vi "GetLocalizedPhraseLowLevel.vi"(7 "Dictionary":T1, 8 "error in (no error)":errorcluster, 10 "Target Language":string, 11 "Key":string) -> (0 "error out":errorcluster, 2 "Key Present?":bool, 3 "Localized Phrase":string)   [LabVIEW 2020]
uses:
  Dictionary--Cluster.ctl
  Font -- Cluster.ctl
  Phrase Dictionary Entry -- Cluster.ctl
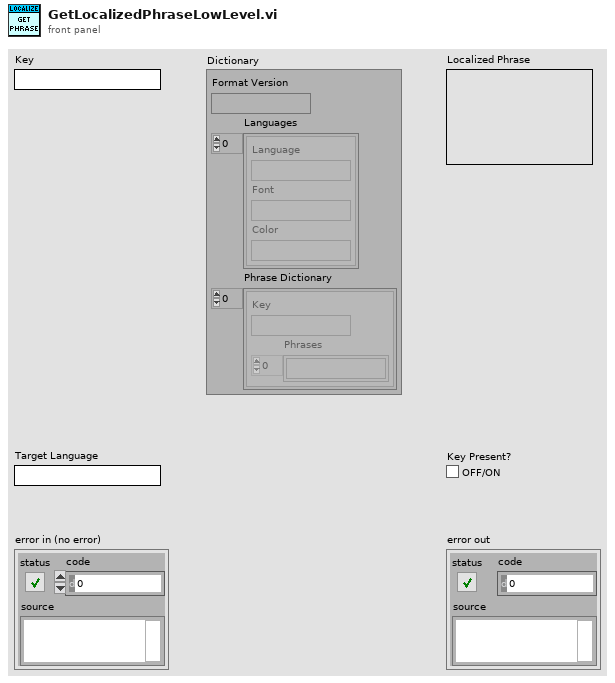
[diagram p1: front panel]
types:
  T1 = typedef "Dictionary--Cluster.ctl" = cluster{"Format Version":string, "Languages":T2[], "Phrase Dictionary":T3[]}
  T2 = typedef "Font -- Cluster.ctl" = cluster{"Language":string, "Font":string, "Color":string}
  T3 = typedef "Phrase Dictionary Entry -- Cluster.ctl" = cluster{"Key":string, "Phrases":string[]}
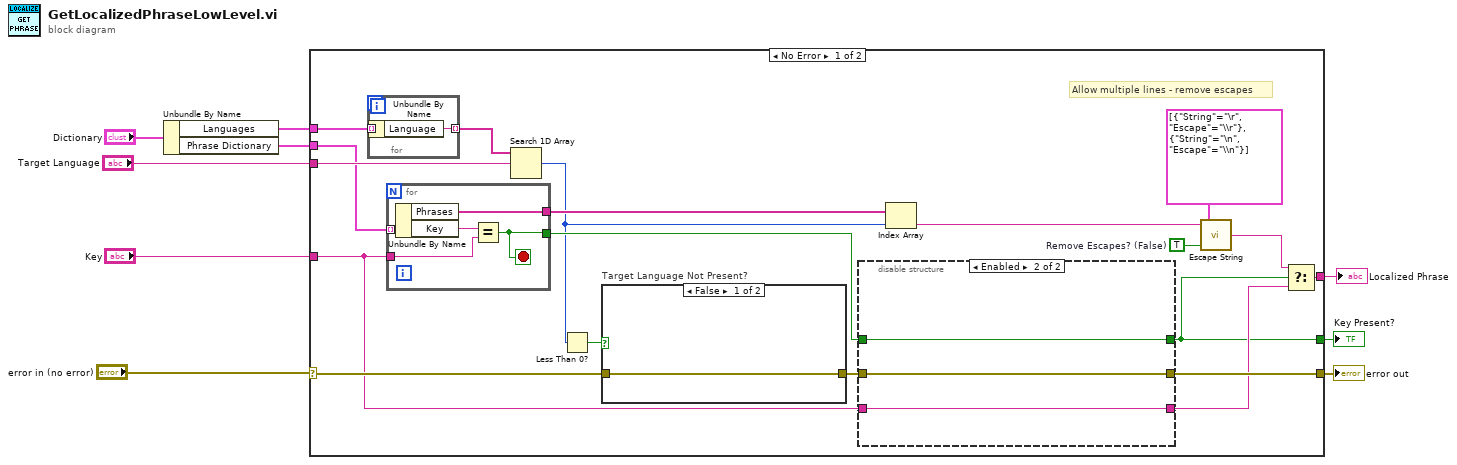
[diagram p0: block diagram]
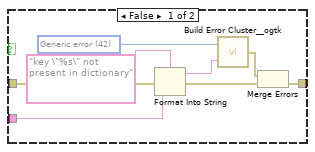
[diagram p3: hidden frame]
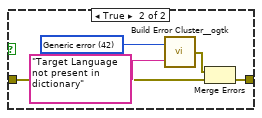
[diagram p4: hidden frame]
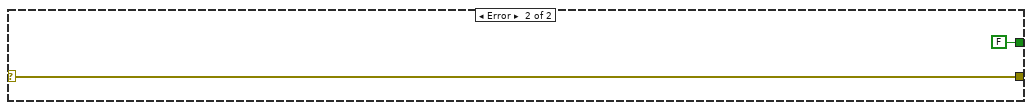
[diagram p5: hidden frame]
diagram:
  n1 = Unbundle By Name("Dictionary") -> ("Languages"=w4:T2[], "Phrase Dictionary"=w2:T3[])
  n2 = case shown="No Error" "error in (no error)" {
    selector: "error in (no error)" -> [w24 w59]
    tunnel: w4 -> [w14 _]
    tunnel: [w16 _] -> w9
    tunnel: [w17 w59] -> w8
    tunnel: "Target Language" -> [w23 _]
    tunnel: "Key" -> [w15 _]
    tunnel: w2 -> [w18 _]
    tunnel: [w10 FALSE] -> w1
    frame No Error {
      w26 = TRUE  # Remove Escapes? (False)
      # "Allow multiple lines - remove escapes"
      n3 = for {
        tunnel: w14 -> [w46] mode=indexing
        tunnel: [w45] -> w13 mode=indexing
        n4 = Unbundle By Name(w46) -> ("Language"=w45:string)
      }
      n5 = for {
        tunnel: w18 -> [w51] mode=indexing
        tunnel: w15 -> [w49]
        tunnel: [w48] -> w21
        tunnel: [w47] -> w22
        stop <- w48 stop-if-true
        n6 = Unbundle By Name(w51) -> ("Phrases"=w47:string[], "Key"=w50:string)
        n7 = Equal?(x=w50, y=w49) -> (x = y?=w48:bool)
      }
      n8 = Search 1D Array(1D array=w13, element=w23) -> (index of element=w20:i32)  [unwired: 1 in]
      n9 = Less Than 0?(x=w20) -> (x < 0?=w28:bool)
      n10 = case "Target Language Not Present?" shown="False" w28 {
        tunnel: w24 -> [w52 w54]
        tunnel: [w52 w53] -> w27
        frame False {
        }
        frame True {
          w57 = 42 items=["No error", "Argument error", "Memory is full", "Out of zone", "End of file", "File already open", "Generic file I/O error", "File not found", "File permission error", "Disk is full", "Duplicate path", "Too many files open", "System feature not enabled", "Resource file not found", "Cannot add resource", "Resource not found", "Image not found", "Image memory error", "Pen does not exist", "Config type invalid", "Config token not found", "Config parse error", "Config memory error", "Bad external code format", "Bad external code offset", "External code not present", "Null window", "Destroy window error", "Null menu", "Print aborted", "Bad print record", "Print driver error", "Windows error during printing", "Memory error during printing", "Print dialog error", "Generic print error", "Invalid device refnum", "Device not found", "Device parameter error", "Device unit error", "Cannot open device", "Device call aborted", "Generic error", "Cancelled by user", "Object ID too low", "Object ID too high", "Object not in heap", "Unknown heap", "Unknown object (invalid DefProc)", "Unknown object (DefProc not in table)", "Message out of range", "Invalid (null) method", "Unknown message", "Manager call not supported", "Bad address", "Network operation in progress", "Network operation timed out", "Connection is busy", "Network attribute not supported", "Network error", "Address in use", "System out of memory", "Connection aborted", "Connection refused", "Not connected", "Already connected", "Connection closed", "Initialization error (interapplication manager)", "Bad occurrence", "Wait on unbound occurrence handler", "Occurrence queue overflow", "Datalog type conflict", "Unused", "Unrecognized type (interapplication manager)", "Memory corrupt", "Failed to make temporary DLL", "Old CIN version", "Drag socket not found", "Failed to load drop-object", "Failed to register OLE object", "Failed to release OLE object", "Format specifier type mismatch", "Unknown format specifier", "Too few format specifiers", "Too many format specifiers", "Scan failed", "Newer CIN version", "Error converting to variant", "Runtime menu error", "Password tampered", "Variant attribute not found", "Incompatible variant data type", "Event data is not available", "Event Store is not present", "Occurrence is not found", "Event Queue is not created", "Event info is not available", "Refnum passed is NULL", "Error retrieving Class GUID", "Error retrieving CoClass GUID", "Error retrieving TypeLib GUID.", "Bad built application magic bytes.", "Specific driver is different from the specific driver associated with the Logical Name.", "There is no session opened to the class driver.", "Max Error", "MAX - Error with config objects", "MAX - Error loading configuration", "MAX - Group not supported"]
          n11 = call <userlib>:"Build Error Cluster__ogtk.vi"("String to Prepend to source (\"\")"="Target Language not present in dictionary" ("String to Prepend to source (\"\")"), "code"=w57) -> ("error out"=w55:errorcluster)
          n12 = Merge Errors(w55, w54) -> (w53:errorcluster)
        }
      }
      n13 = disable-structure shown="Enabled" {
        disable-tunnel: w27 -> [w32 w44]
        disable-tunnel: w21 -> [w31 w43]
        disable-tunnel: [w30 w44] -> w17
        disable-tunnel: w15 -> [w29 w42]
        disable-tunnel: [_ w43] -> w10
        disable-tunnel: [_ w42] -> w11
        frame Disabled {
          n14 = case "Key Present?" shown="True" w31 {
            tunnel: w32 -> [w37 w41]
            tunnel: [w38 w41] -> w30
            tunnel: w29 -> [w34 _]
            frame False {
              w40 = 42 items=["No error", "Argument error", "Memory is full", "Out of zone", "End of file", "File already open", "Generic file I/O error", "File not found", "File permission error", "Disk is full", "Duplicate path", "Too many files open", "System feature not enabled", "Resource file not found", "Cannot add resource", "Resource not found", "Image not found", "Image memory error", "Pen does not exist", "Config type invalid", "Config token not found", "Config parse error", "Config memory error", "Bad external code format", "Bad external code offset", "External code not present", "Null window", "Destroy window error", "Null menu", "Print aborted", "Bad print record", "Print driver error", "Windows error during printing", "Memory error during printing", "Print dialog error", "Generic print error", "Invalid device refnum", "Device not found", "Device parameter error", "Device unit error", "Cannot open device", "Device call aborted", "Generic error", "Cancelled by user", "Object ID too low", "Object ID too high", "Object not in heap", "Unknown heap", "Unknown object (invalid DefProc)", "Unknown object (DefProc not in table)", "Message out of range", "Invalid (null) method", "Unknown message", "Manager call not supported", "Bad address", "Network operation in progress", "Network operation timed out", "Connection is busy", "Network attribute not supported", "Network error", "Address in use", "System out of memory", "Connection aborted", "Connection refused", "Not connected", "Already connected", "Connection closed", "Initialization error (interapplication manager)", "Bad occurrence", "Wait on unbound occurrence handler", "Occurrence queue overflow", "Datalog type conflict", "Unused", "Unrecognized type (interapplication manager)", "Memory corrupt", "Failed to make temporary DLL", "Old CIN version", "Drag socket not found", "Failed to load drop-object", "Failed to register OLE object", "Failed to release OLE object", "Format specifier type mismatch", "Unknown format specifier", "Too few format specifiers", "Too many format specifiers", "Scan failed", "Newer CIN version", "Error converting to variant", "Runtime menu error", "Password tampered", "Variant attribute not found", "Incompatible variant data type", "Event data is not available", "Event Store is not present", "Occurrence is not found", "Event Queue is not created", "Event info is not available", "Refnum passed is NULL", "Error retrieving Class GUID", "Error retrieving CoClass GUID", "Error retrieving TypeLib GUID.", "Bad built application magic bytes.", "Specific driver is different from the specific driver associated with the Logical Name.", "There is no session opened to the class driver.", "Max Error", "MAX - Error with config objects", "MAX - Error loading configuration", "MAX - Group not supported"]
              n15 = Format Into String(format string="key \"%s\" not present in dictionary" ("String to Prepend to source (\"\")"), error in=w37, w34) -> (resulting string=w33:string, error out=w36:errorcluster)  [unwired: 1 in]
              n16 = call <userlib>:"Build Error Cluster__ogtk.vi"("String to Prepend to source (\"\")"=w33, "code"=w40) -> ("error out"=w39:errorcluster)
              n17 = Merge Errors(w39, w36) -> (w38:errorcluster)
            }
            frame True {
            }
          }
        }
        frame Enabled {
        }
      }
      n18 = Index Array(array=w22, index=w20) -> (element=w19:string)
      n19 = call <vilib>:"Escape String.vi"("Remove Escapes? (False)"=w26, "Escapes"=cluster{"String":string, "Escape":string}[] [{"String"="\r", "Escape"="\\r"}, {"String"="\n", "Escape"="\\n"}], "String in"=w19) -> ("String out"=w12:string)
      n20 = Select(t=w12, s=w10, f=w11) -> (s? t:f=w16:string)
    }
    frame Error {
    }
  }
  "Localized Phrase" <- w9
  "error out" <- w8
  "Key Present?" <- w1
